vi "currentQuadrant.vi"(11 "Wheel":dbl) -> (3 "Quadrent":dbl)   [LabVIEW 2011]
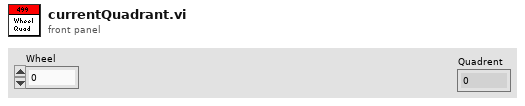
[diagram p1: front panel]
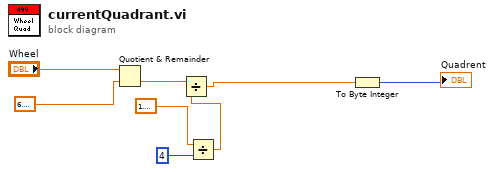
[diagram p0: block diagram]
diagram:
  n1 = Quotient & Remainder(x="Wheel", y=6.283185307179586) -> (floor(x/y)=w6:dbl)  [unwired: 1 out]
  n2 = Divide(x=1.5707963267948966, y=4) -> (x/y=w1:dbl)
  n3 = Divide(x=w6, y=w1) -> (x/y=w4:dbl)
  n4 = To Byte Integer(number=w4) -> (8bit integer=→"Quadrent":i8)
